vi "Dynamixel U32 to I32.vi"(0 "U32 In":u32, 1 "Function":T1) -> (5 "I32 Out":i32)   [LabVIEW 2022 SP3]
uses:
  Dynamixel Commands.ctl
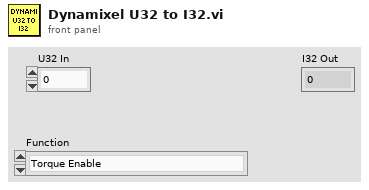
[diagram p1: front panel]
types:
  T1 = typedef "Dynamixel Commands.ctl" = enum16{"Torque Enable", "Present Position", "Threshold", "Max Position Limit", "Acceleration Profile", "Velocity Profile", "Goal Position", "Position Proportional Gain", "Position Integral Gain", "Position Differential Gain ", "Shutdown", "Write Operating Mode", "Read Operating Mode"}
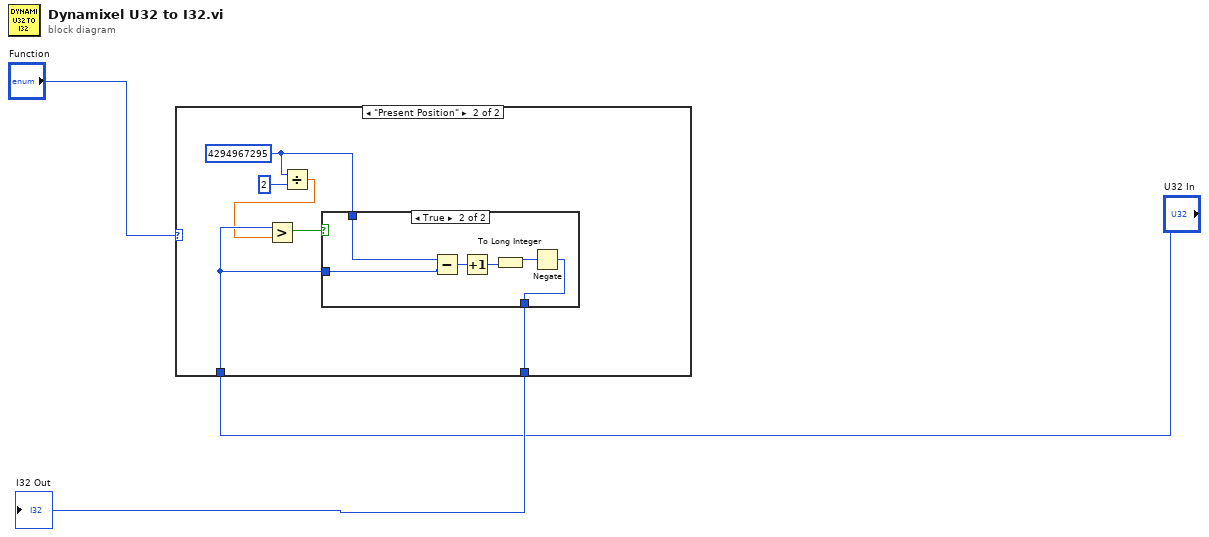
[diagram p0: block diagram]
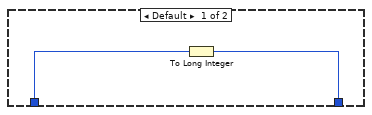
[diagram p2: hidden frame]
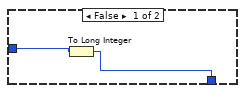
[diagram p3: hidden frame]
diagram:
  n1 = case shown="\"Present Position\"" "Function" {
    tunnel: "U32 In" -> [w5 w10]
    tunnel: [w4 w11] -> w3
    frame Default {
      n2 = To Long Integer(number=w5) -> (32bit integer=w4:i32)
    }
    frame "Present Position" {
      w9 = u32 4294967295 ("y")
      n3 = Divide(x=w9, y=u32 2) -> (x/y=w7:dbl)
      n4 = Greater?(x=w10, y=w7) -> (0:w6:bool)
      n5 = case shown="True" w6 {
        tunnel: w10 -> [w13 w19]
        tunnel: [w12 w15] -> w11
        tunnel: w9 -> [_ w14]
        frame False {
          n6 = To Long Integer(number=w13) -> (32bit integer=w12:i32)
        }
        frame True {
          n7 = Subtract(x=w14, y=w19) -> (x-y=w18:u32)
          n8 = Increment(x=w18) -> (x+1=w17:u32)
          n9 = To Long Integer(number=w17) -> (32bit integer=w16:i32)
          n10 = Negate(x=w16) -> (-x=w15:i32)
        }
      }
    }
  }
  "I32 Out" <- w3
